vi "Format String.vi"() -> ()   [LabVIEW 2011]
panel:
  out "output 1":i32
  out "resulting string":string
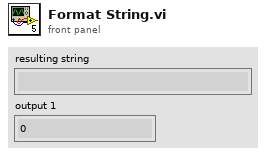
[diagram p1: front panel]
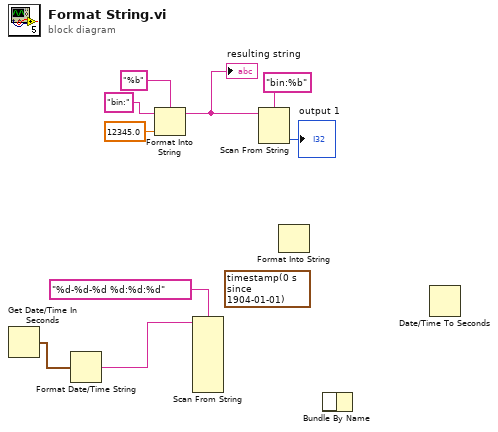
[diagram p0: block diagram]
diagram:
  (unwired) timestamp(0 s since 1904-01-01) ("current time")
  n1 = Get Date/Time In Seconds() -> (seconds since 1Jan1904=w2:timestamp)
  n2 = Format Date/Time String(seconds (now)=w2) -> (date/time string=w1:string)  [unwired: 2 in]
  n3 = Format Into String(format string="%b", initial string="bin:", 12345.0 ("input 1")) -> (resulting string=w7:string)  [unwired: 1 in, 1 out]
  "resulting string" <- w7
  n4 = Scan From String(format string="%d-%d-%d %d:%d:%d", input string=w1) -> ()  [unwired: 14 in, 3 out]
  n5 = Scan From String(format string="bin:%b", input string=w7) -> (output 1=→"output 1":i32)  [unwired: 3 in, 3 out]
  n6 = Format Into String() -> ()  [unwired: 4 in, 2 out]
  n7 = Bundle By Name() -> ()  [unwired: 2 in, 1 out]
  n8 = Date/Time To Seconds() -> ()  [unwired: 2 in, 1 out]
